vi "Format.vi"(8 "error in (no error)":errorcluster, 10 "log record":T1 {"timestamp" format="%<%x %.3X>T"}, 11 "JSON in":refnum<class "JSON.lvclass">) -> (0 "error out":errorcluster, 2 "log line":string, 3 "JSON out":refnum<class "JSON.lvclass">)   [LabVIEW 2018, in "Logging.lvlib" / "JSON.lvclass"]
uses:
  JSON.lvclass
  Log Record.ctl
  Logger/Internal Log Levels.ctl
  <vilib>/addons/_JKI.lib/Serialization/JSON/Library/Timestamp Options.ctl
  JSON.lvclass/JSON.ctl
  <vilib>/addons/_JKI.lib/Serialization/JSON/JKI JSON Serialization.lvlib
  Logging.lvlib
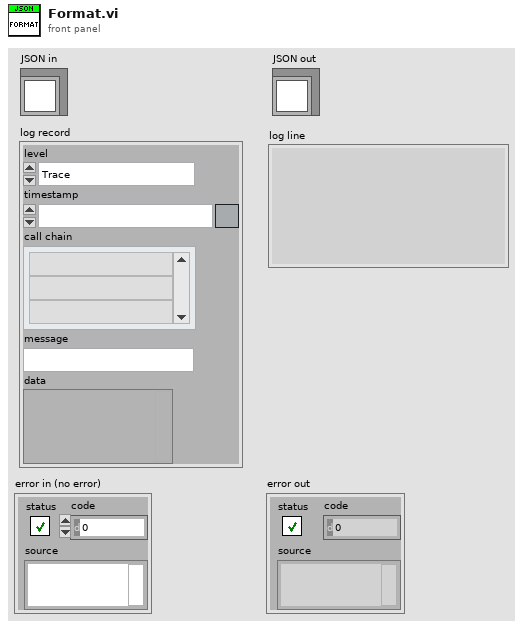
[diagram p1: front panel]
types:
  T1 = typedef "Logging.lvlib/Log Record.ctl" = cluster{"level":T2, "timestamp":timestamp, "call chain":string[], "message":string, "data":variant}
  T2 = typedef "Logging.lvlib/Internal Log Levels.ctl" = enum16{"Trace", "Debug", "Info", "Warning", "Error", "Critical", "Internal"}
  T3 = typedef "JKI JSON Serialization.lvlib/Timestamp Options.ctl" = cluster{"Convert Timestamps":bool, "UTC":bool}
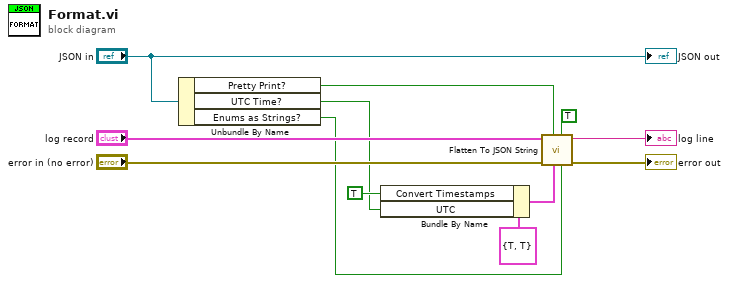
[diagram p0: block diagram]
diagram:
  n1 = Unbundle By Name("JSON in") -> ("Pretty Print?"=w3:bool, "UTC Time?"=w2:bool, "Enums as Strings?"=w1:bool)
  n2 = Bundle By Name(cluster=T3 {"Convert Timestamps"=TRUE, "UTC"=TRUE} ("Timestamp Options"), "Convert Timestamps"=TRUE, "UTC"=w2) -> (w5:T3)
  n3 = call <vilib>:"Flatten To JSON String.vi"("Enums As String (F)"=w1, "Numeric Extensions (F)"=TRUE, "Timestamp Options"=w5, "Multiline (T)"=w3, "error in (no error)"="error in (no error)", "Variant"="log record") -> ("error out"=→"error out":errorcluster, "JSON String"=→"log line":string)  [unwired: 4 in]
  "JSON out" <- "JSON in"
